vi "Disconnect.vi"(7 "error in (no error)":errorcluster, 10 "GenericCanAdapterClass in":refnum<class "GenericCanAdapterClass.lvclass">) -> (0 "error out":errorcluster, 3 "GenericCanAdapterClass out":refnum<class "GenericCanAdapterClass.lvclass">)   [LabVIEW 2011, in "GenericCanAdapterClass.lvclass"]
uses:
  GenericCanAdapterClass.lvclass
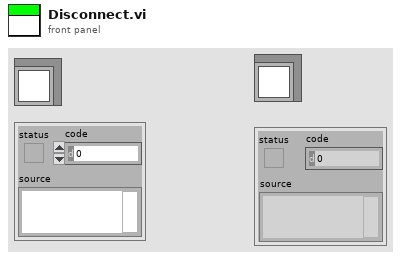
[diagram p1: front panel]
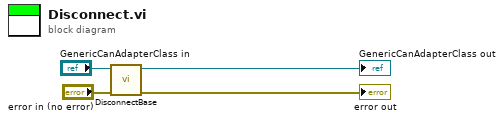
[diagram p0: block diagram]
diagram:
  n1 = call-dynamic "DisconnectBase.vi"("error in (no error)"="error in (no error)", "GenericCanAdapterClass in"="GenericCanAdapterClass in") -> ("error out"=→"error out":errorcluster, "GenericCanAdapterClass out"=→"GenericCanAdapterClass out":refnum<class "GenericCanAdapterClass.lvclass">)  [unwired: 8 in]
